vi "waitTarget-XY.vi"(0 "Device in X":refnum<k24>, 5 "GetPOS X":refnum<vi>, 7 "Position X":sgl, 9 "GetPOS Y":refnum<vi>, 11 "Device in Y":refnum<k24>, 12 "Position Y":sgl) -> (4 "Device out X":refnum<k24>, 6 "GetPOS X":dbl format="%#_6f", 8 "GetPOS Y":dbl format="%#_6f", 15 "Device out Y":refnum<k24>)   [LabVIEW 2014]
doc: "André Romero - 2018\nandretec@ifsc.usp.br"
uses:
  C:/user-Lab/AndreTec/GITs/andretec/Thorlabs-Vector-Move/kinesisTec/Kinesis/Thorlabs.MotionControl.TCube.DCServoCLI.dll
  kinesisTec/Kinesis/Thorlabs.MotionControl.TCube.DCServoCLI.dll
panel:
  in  "error":dbl=0.004 format="%#_13g"
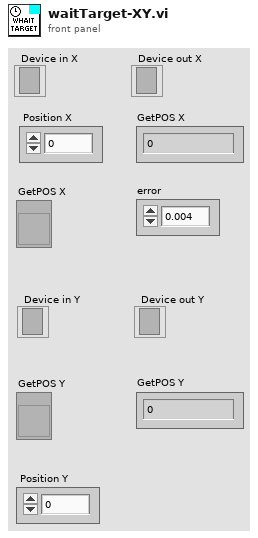
[diagram p1: front panel]
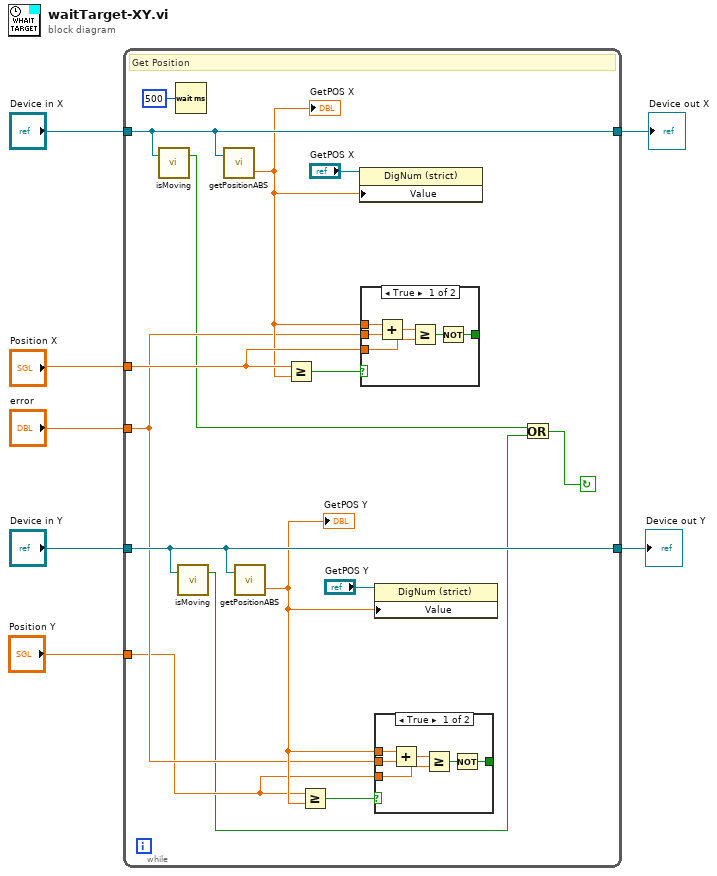
[diagram p0: block diagram]
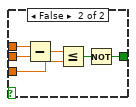
[diagram p2: hidden frame]
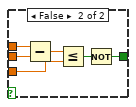
[diagram p3: hidden frame]
diagram:
  n1 = while {
    tunnel: "Device in X" -> [w22]
    tunnel: [w22] -> w6
    tunnel: "Position X" -> [w18]
    tunnel: "error" -> [w12]
    tunnel: "Device in Y" -> [w15]
    tunnel: [w15] -> w2
    tunnel: "Position Y" -> [w11]
    stop <- w10 continue-if-true
    # "Get Position"
    n2 = call "isMoving.vi"("Device in"=w22) -> ("IsMoving"=w9:bool)  [unwired: 1 in, 1 out]
    n3 = Wait (ms)(milliseconds to wait=u32 500) -> ()  [unwired: 1 out]
    n4 = call "isMoving.vi"("Device in"=w15) -> ("IsMoving"=w8:bool)  [unwired: 1 in, 1 out]
    n5 = call "getPositionABS.vi"("Device"=w22) -> ("GetPOS"=w17:dbl)  [unwired: 1 in, 1 out]
    "GetPOS X" <- w17
    n6 = call "getPositionABS.vi"("Device"=w15) -> ("GetPOS"=w13:dbl)  [unwired: 1 in, 1 out]
    "GetPOS Y" <- w13
    n7 = Greater Or Equal?(x=w18, y=w17) -> (x >= y?=w19:bool)
    n8 = Greater Or Equal?(x=w11, y=w13) -> (x >= y?=w14:bool)
    n9 = property class="DigNum (strict)"(reference="GetPOS X", "Value"=w17) -> ()  [unwired: 1 in, 2 out]
    n10 = case shown="True" w19 {
      tunnel: w17 -> [w40 w46]
      tunnel: w12 -> [w39 w45]
      tunnel: w18 -> [w37 w43]
      tunnel: [w35 w41] -> _
      frame True {
        n11 = Add(x=w40, y=w39) -> (x+y=w38:dbl)
        n12 = Greater Or Equal?(x=w38, y=w37) -> (x >= y?=w36:bool)
        n13 = Not(x=w36) -> (.not. x?=w35:bool)
      }
      frame False {
        n14 = Subtract(x=w46, y=w45) -> (x-y=w44:dbl)
        n15 = Less Or Equal?(x=w44, y=w43) -> (x <= y?=w42:bool)
        n16 = Not(x=w42) -> (.not. x?=w41:bool)
      }
    }
    n17 = property class="DigNum (strict)"(reference="GetPOS Y", "Value"=w13) -> ()  [unwired: 1 in, 2 out]
    n18 = case shown="True" w14 {
      tunnel: w13 -> [w28 w34]
      tunnel: w12 -> [w27 w33]
      tunnel: w11 -> [w25 w31]
      tunnel: [w23 w29] -> _
      frame True {
        n19 = Add(x=w28, y=w27) -> (x+y=w26:dbl)
        n20 = Greater Or Equal?(x=w26, y=w25) -> (x >= y?=w24:bool)
        n21 = Not(x=w24) -> (.not. x?=w23:bool)
      }
      frame False {
        n22 = Subtract(x=w34, y=w33) -> (x-y=w32:dbl)
        n23 = Less Or Equal?(x=w32, y=w31) -> (x <= y?=w30:bool)
        n24 = Not(x=w30) -> (.not. x?=w29:bool)
      }
    }
    n25 = Or(x=w9, y=w8) -> (x .or. y?=w10:bool)
  }
  "Device out X" <- w6
  "Device out Y" <- w2
